vi "Pre Launch Init.vi"(11 "LeakyViewable in":refnum<class "LeakyViewable.lvclass">) -> (0 "error out":errorcluster, 3 "LeakyViewable out":refnum<class "LeakyViewable.lvclass">)   [LabVIEW 2017, in "LeakyViewable.lvlib" / "LeakyViewable.lvclass"]
doc: "(<B>Filename</B>: Actor Framework.lvlib:Actor.lvclass:Pre Launch Init.vi)\n\nDefines behavior that occurs after the Launch Nested Actor method is invoked but before the actor's Actor Core method begins running.\n\nBy default, this method does nothing. A descendant class may override it to define behavior."
uses:
  LeakyViewable.lvclass
  Leak Location.ctl
  Source/IViewable/IViewable/IViewable.lvclass
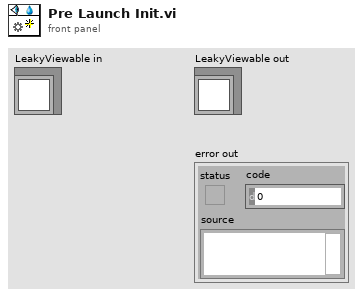
[diagram p1: front panel]
types:
  T1 = typedef "LeakyViewable.lvlib/LeakyViewable.lvclass/Leak Location.ctl" = enum16{"Pre Launch Init", "Entering Actor Core", "Actor Core", "Exiting Actor Core", "Stop Core", "Handle Error"}
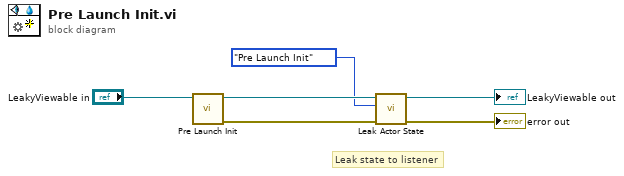
[diagram p0: block diagram]
diagram:
  # "Leak state to listener"
  n1 = call-parent "Pre Launch Init.vi"("IViewable in"="LeakyViewable in") -> ("error out"=w6:errorcluster, "IViewable out"=w3:refnum<class "LeakyViewable.lvclass">)  [unwired: 9 in]
  n2 = call "Leak Actor State.vi"("error in (no error)"=w6, "Location"=Leak_Location."Pre Launch Init", "ViewableOne in"=w3) -> ("error out"=→"error out":errorcluster, "ViewableOne out"=→"LeakyViewable out":refnum<class "LeakyViewable.lvclass">)  [unwired: 7 in]
